vi "Main.vi"() -> ()   [LabVIEW 2018, in "PrototypePatternDemo.lvclass"]
uses:
  PrototypePatternDemo.lvclass
  ConsoleOut/Print Options.ctl
  BundledShapeCache Class/BundledShapeCache.lvclass
  Shape Class/pShape.lvclass
panel:
  out "error out":errorcluster
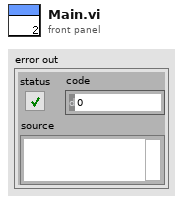
[diagram p1: front panel]
types:
  T1 = typedef "Print Options.ctl" = enum16{"Create", "Get Reference", "Print", "Print Header", "Close"}
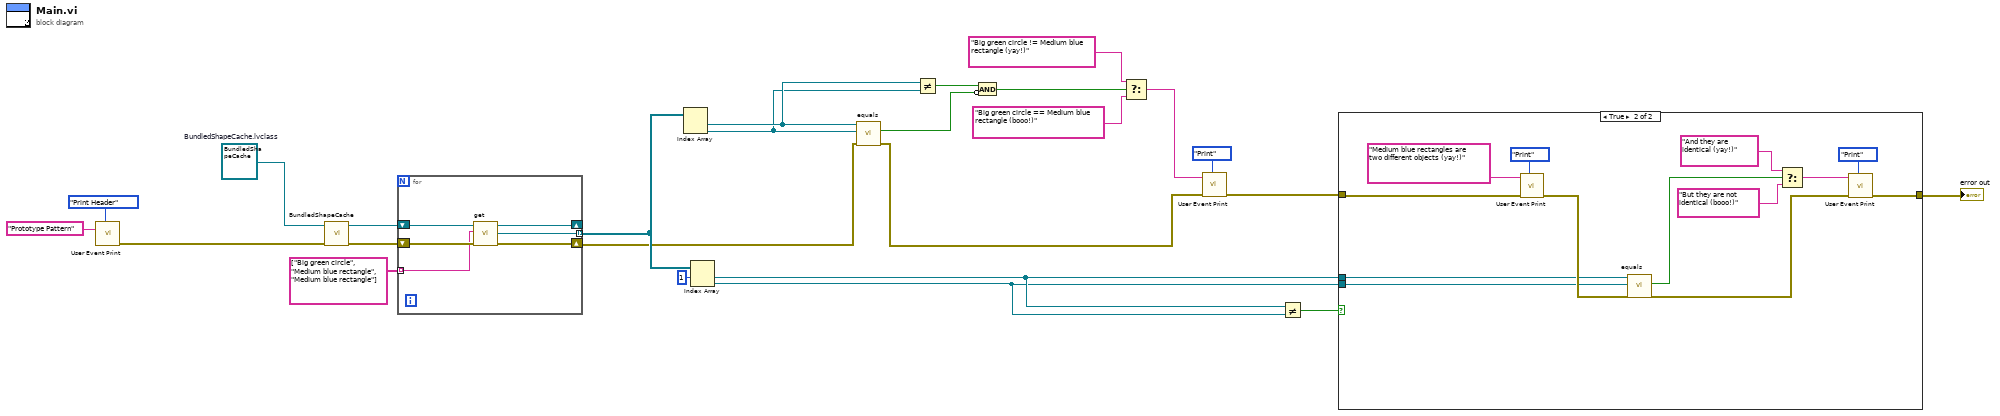
[diagram p0: block diagram]
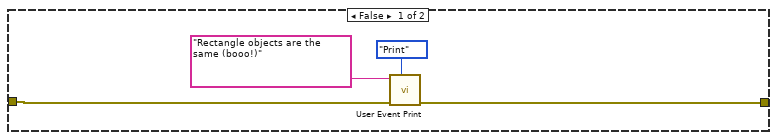
[diagram p2: hidden frame]
diagram:
  w22 = refnum<class "BundledShapeCache.lvclass"> refnum  # BundledShapeCache.lvclass
  n1 = call "User Event Print.vi"("Options"=Print_Options."Print Header", "String to Print"="Prototype Pattern") -> ("error out"=w25:errorcluster)  [unwired: 8 in, 1 out]
  n2 = call "BundledShapeCache.vi"("error in (no error)"=w25, "BundledShapeCache in"=w22) -> ("error out"=w21:errorcluster, "BundledShapeCache out"=w20:refnum<class "BundledShapeCache.lvclass">)  [unwired: 8 in]
  n3 = for {
    tunnel: [w27] -> w9 mode=indexing
    shift-right: [w29] -> w5
    shift-left: w21 -> [w31]
    shift-right: [w30] -> _
    shift-left: w20 -> [w28]
    tunnel: string[] ["Big green circle", "Medium blue rectangle", "Medium blue rectangle"] ("Key") -> [w26] mode=indexing
    n4 = call "get.vi"("error in (no error)"=w31, "Key"=w26, "BundledShapeCache in"=w28) -> ("error out"=w29:errorcluster, "pShape.lvclass"=w27:refnum<class "pShape.lvclass">, "BundledShapeCache out"=w30:refnum<class "BundledShapeCache.lvclass">)  [unwired: 6 in]
  }
  n5 = Index Array(array=w9) -> (element #1=w11:refnum<class "pShape.lvclass">, element #2=w10:refnum<class "pShape.lvclass">)  [unwired: 2 in]
  n6 = Index Array(array=w9, index #1=1 ("index")) -> (element #1=w7:refnum<class "pShape.lvclass">, element #2=w6:refnum<class "pShape.lvclass">)  [unwired: 1 in]
  n7 = call-dynamic "equals.vi"("error in (no error)"=w5, "object 2"=w10, "pShape in"=w11) -> ("error out"=w4:errorcluster, "equal?"=w2:bool)  [unwired: 6 in, 1 out]
  n8 = Not Equal?(x=w11, y=w10) -> (x != y?=w3:bool)
  n9 = Compound Arithmetic op=AND(w3, invert w2) -> (w18:bool)
  n10 = Select(t="Big green circle != Medium blue rectangle (yay!)", s=w18, f="Big green circle == Medium blue rectangle (booo!)") -> (s? t:f=w16:string)
  n11 = call "User Event Print.vi"("Options"=Print_Options."Print", "error in (no error)"=w4, "String to Print"=w16) -> ("error out"=w13:errorcluster)  [unwired: 7 in, 1 out]
  n12 = Not Equal?(x=w7, y=w6) -> (x != y?=w14:bool)
  n13 = case shown="True" w14 {
    tunnel: w13 -> [w33 w38]
    tunnel: w7 -> [_ w40]
    tunnel: w6 -> [_ w39]
    tunnel: [w32 w36] -> w1
    frame False {
      n14 = call "User Event Print.vi"("Options"=Print_Options."Print", "error in (no error)"=w33, "String to Print"="Rectangle objects are the same (booo!)") -> ("error out"=w32:errorcluster)  [unwired: 7 in, 1 out]
    }
    frame True {
      n15 = call "User Event Print.vi"("Options"=Print_Options."Print", "error in (no error)"=w38, "String to Print"="Medium blue rectangles are two different objects (yay!)") -> ("error out"=w46:errorcluster)  [unwired: 7 in, 1 out]
      n16 = call-dynamic "equals.vi"("error in (no error)"=w46, "object 2"=w39, "pShape in"=w40) -> ("error out"=w37:errorcluster, "equal?"=w43:bool)  [unwired: 6 in, 1 out]
      n17 = Select(t="And they are identical (yay!)", s=w43, f="But they are not identical (booo!)") -> (s? t:f=w44:string)
      n18 = call "User Event Print.vi"("Options"=Print_Options."Print", "error in (no error)"=w37, "String to Print"=w44) -> ("error out"=w36:errorcluster)  [unwired: 7 in, 1 out]
    }
  }
  "error out" <- w1
